vi "Bit Shift In.vi"(7 "reset":bool, 9 "shift index":bool, 10 "sample bit":bool, 11 "data bit in":bool) -> (3 "sample":u32)   [LabVIEW 2013, in "I2S-TDM.lvlib"]
uses:
  I2S-TDM.lvlib
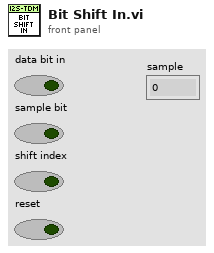
[diagram p1: front panel]
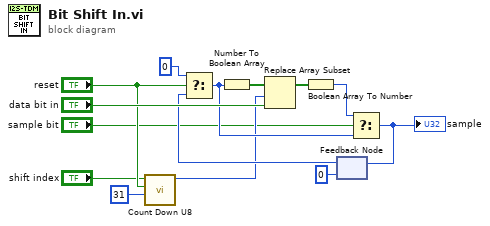
[diagram p0: block diagram]
diagram:
  n1 = call "Count Down U8.vi"("reset value"=u8 31, "reset"="reset", "decrement"="shift index") -> ("count"=w4:u8)  [unwired: 8 in]
  n2 = feedback #1(u32 0) -> (w6:u32)
  n3 = Select(t=u32 0, s="reset", f=w6) -> (s? t:f=w7:u32)
  n4 = Number To Boolean Array(number=w7) -> (Boolean array=w12:bool[])
  n5 = Replace Array Subset(array=w12, new element="data bit in", index=w4) -> (w11:bool[])
  n6 = Boolean Array To Number(Boolean array=w11) -> (number=w9:u32)
  n7 = Select(t=w9, s="sample bit", f=w7) -> (s? t:f=w8:u32)
  "sample" <- w8
  n8 = feedback-in #1(w8) -> ()
